vi "图片读取与保存.vi"() -> ()   [LabVIEW 2020]
panel:
  in  "Image Type":T1 items=["Grayscale (U8)", "Grayscale (I16)", "Grayscale (SGL)", "Complex (CSG)", "RGB (U32)", "HSL (U32)", "RGB (U64)", "Grayscale (U16)"]
  in  "停止":bool
  out "Image":T2(plugin-control)
  out "error out":errorcluster
  out "布尔":bool
  in  "File Path":path
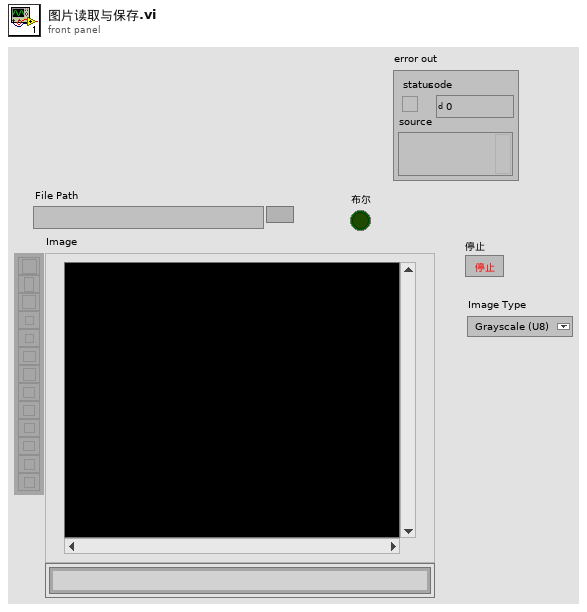
[diagram p1: front panel]
types:
  T1 = typedef "Image Type" = u32
  T2 = typedef "IMAQ Image.ctl" = refnum<image>
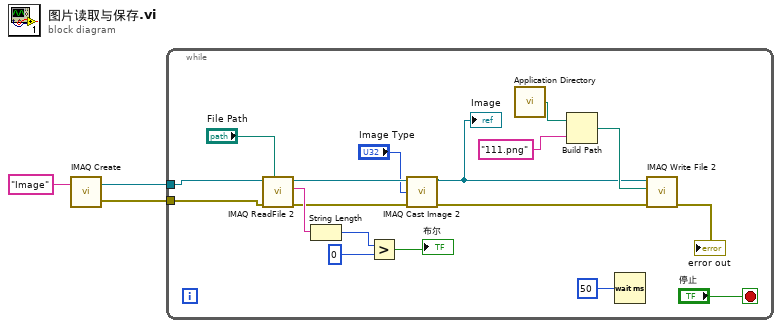
[diagram p0: block diagram]
diagram:
  n1 = call "IMAQ Create"("Image Name"="Image") -> ("New Image"=w2:T2, "error out"=w1:errorcluster)  [unwired: 4 in]
  n2 = while {
    tunnel: w2 -> [w10]
    tunnel: w1 -> [w9]
    stop <- "停止" stop-if-true
    n3 = call "IMAQ ReadFile 2"("File Path"="File Path", "error in (no error)"=w9, "Image"=w10) -> ("error out"=w8:errorcluster, "File Type out"=w20:string, "Image Out"=w6:T2)  [unwired: 4 in, 2 out]
    n4 = String Length(string=w20) -> (length=w19:i32)
    n5 = Greater?(x=w19, y=0) -> (0:→"布尔":bool)
    n6 = call "IMAQ Cast Image 2"("Image Src"=w6, "Image Type"="Image Type", "error in (no error)"=w8) -> ("Image Dst Out"=w5:T2, "error out"=w7:errorcluster)  [unwired: 11 in]
    "Image" <- w5
    n7 = call <vilib>:"Application Directory.vi"() -> ("Application Directory"=w16:path)
    n8 = Build Path(base path=w16, name or relative path="111.png") -> (appended path=w14:path)
    n9 = Wait (ms)(milliseconds to wait=u32 50 ("等待时间（毫秒）")) -> ()  [unwired: 1 out]
    n10 = call-poly "IMAQ Write File 2"("error in (no error)"=w7, "File Path"=w14, "Image"=w5) -> ("error out"=→"error out":errorcluster)  [unwired: 7 in, 1 out]
  }
